vi "Keyboard Diagnostics.vi"() -> (0 "error out":errorcluster, 1 "Test Data":T1 {"Numeric Measurement" format="%.2f"})   [LabVIEW 2012]
uses:
  <vilib>/addons/TestStand/_TSLegacy.llb/LabVIEW Test - Test Data.ctl
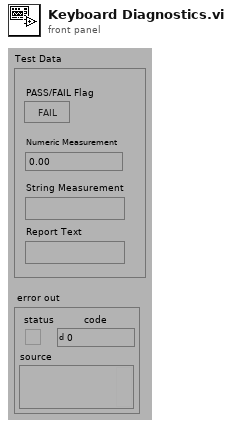
[diagram p1: front panel]
types:
  T1 = typedef "LabVIEW Test - Test Data.ctl" = cluster{"PASS/FAIL Flag":bool, "Numeric Measurement":dbl, "String Measurement":string, "Report Text":string}
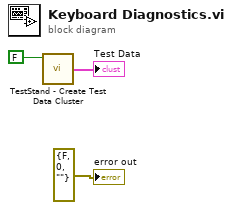
[diagram p0: block diagram]
diagram:
  n1 = call "TestStand - Create Test Data Cluster.vi"("PASS/FAIL Flag"=FALSE) -> ("Test Data"=→"Test Data":T1)  [unwired: 3 in]
  "error out" <- errorcluster {"status"=FALSE, "code"=0, "source"=""} ("error out")
